vi "formatstringtime.vi"(10 "枚举":T1(ring), 11 "字符串":string) -> (3 "result string":string)   [LabVIEW 2016, in "212format_work.lvclass"]
uses:
  212format_work.lvclass
panel:
  out "输出 1":timestamp
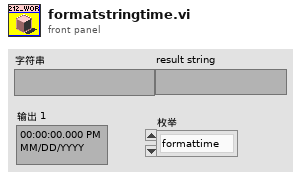
[diagram p1: front panel]
types:
  T1 = enum16{"formattime", "formatminute", "formathour"}
  T2 = typedef "LVDateTimeRec.ctl" = cluster{"秒数的小数部分":dbl, "秒":i32, "分":i32, "时":i32, "日":i32, "月":i32, "年":i32, "天数（周）":i32, "天数（年）":i32, "DST":i32}
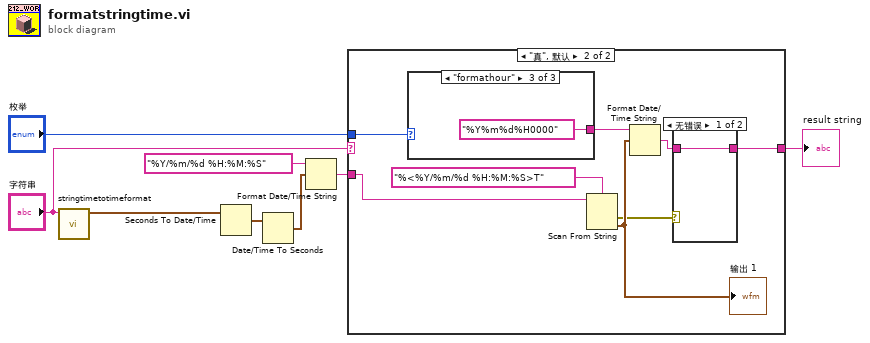
[diagram p0: block diagram]
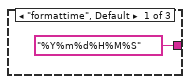
[diagram p3: hidden frame]
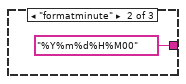
[diagram p4: hidden frame]
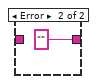
[diagram p5: hidden frame]
diagram:
  n1 = call "stringtimetotimeformat.vi"("data[0]"="字符串") -> ("time stamp"=w6:timestamp)  [unwired: 10 in]
  n2 = Seconds To Date/Time(time stamp (now)=w6) -> (date time rec=w7:T2)  [unwired: 1 in]
  n3 = Date/Time To Seconds(2:w7) -> (0:w5:timestamp)  [unwired: 1 in]
  n4 = Format Date/Time String(time format string (%c)="%Y/%m/%d %H:%M:%S" ("时间格式字符串(%c)"), seconds (now)=w5) -> (date/time string=w3:string)  [unwired: 1 in]
  n5 = case shown="\"真\", 默认" "字符串" {
    selector: "字符串" -> [w9 _]
    tunnel: w3 -> [_ w17]
    tunnel: [w9 w11] -> w8
    tunnel: "枚举" -> [_ w10]
    frame "" {
    }
    frame "真", Default {
      n6 = case shown="\"formathour\"" w10 {
        tunnel: ["%Y%m%d%H%M%S" ("时间格式字符串(%c)") "%Y%m%d%H%M00" ("时间格式字符串(%c)") "%Y%m%d%H0000" ("时间格式字符串(%c)")] -> w15
        frame "formattime", Default {
        }
        frame "formatminute" {
        }
        frame "formathour" {
        }
      }
      n7 = Scan From String(format string="%<%Y/%m/%d %H:%M:%S>T" ("格式字符串"), input string=w17) -> (error out=w13:errorcluster, output 1=w16:timestamp)  [unwired: 3 in, 2 out]
      "输出 1" <- w16
      n8 = Format Date/Time String(time format string (%c)=w15, seconds (now)=w16) -> (date/time string=w12:string)  [unwired: 1 in]
      n9 = case shown="无错误" w13 {
        tunnel: [w21 "" ("date/time string")] -> w11
        tunnel: w12 -> [w21 _]
        frame No Error {
        }
        frame Error {
        }
      }
    }
  }
  "result string" <- w8
